vi "Number Widget.vi"(8 "Error In":errorcluster, 11 "Post-Bundled Subclass":refnum<class "4. Number Widget.lvclass">) -> (0 "Error Out":errorcluster, 3 "New Number Widget":refnum<class "4. Number Widget.lvclass">)   [LabVIEW 2013, in "4. Number Widget.lvclass"]
doc: "Copyright (c) 2016 Sze Howe Koh\nThis code is licensed under the MIT license"
uses:
  4. Number Widget.lvclass
  src/LabVIEW/Qt Widgets/QBoxLayout/Direction.ctl
  src/LabVIEW/Qt Widgets/QFrame/Shadow.ctl
  src/LabVIEW/Qt Widgets/QFrame/Shape.ctl
  4. Number Widget.lvclass/4. Number Widget.ctl
  src/LabVIEW/LQ Core/LQCoreEngine/_Polymorphic Instances/Connect_SignatureIn_QtSlot.vi
  src/LabVIEW/Qt Widgets/QFrame/setFrameShadow.vi
  src/LabVIEW/Qt Widgets/QFrame/setFrameShape.vi
  src/LabVIEW/Qt Widgets/QLCDNumber/QLCDNumber.lvclass
  src/LabVIEW/Qwt/QwtSlider/QwtSlider.lvclass
  src/LabVIEW/Qt Widgets/QBoxLayout/QBoxLayout.lvclass
  src/LabVIEW/Qt Widgets/QWidget/QWidget.lvclass
  src/LabVIEW/LQ Core/LQCoreEngine/LQCoreEngine.lvclass
  src/LabVIEW/Qt Widgets/QFrame/QFrame.lvclass
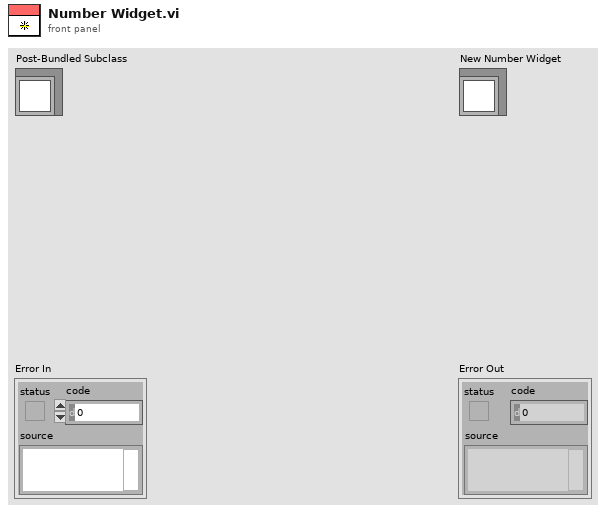
[diagram p1: front panel]
types:
  T1 = typedef "QFrame.lvclass/Shape.ctl" = i32
  T2 = typedef "QFrame.lvclass/Shadow.ctl" = i32
  T3 = typedef "QBoxLayout.lvclass/Direction.ctl" = i32
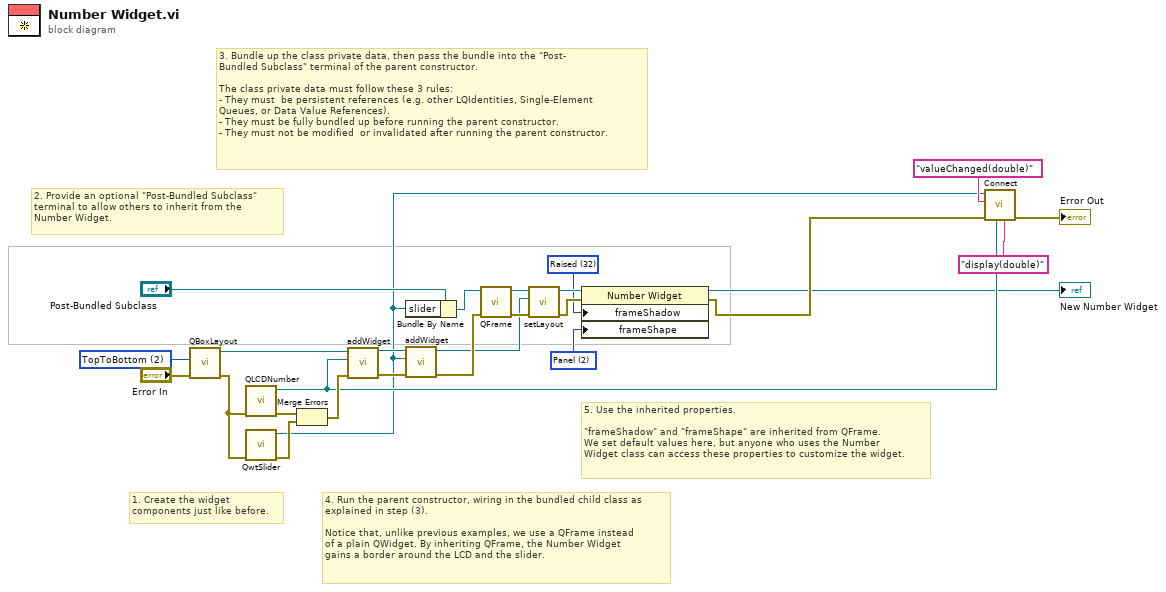
[diagram p0: block diagram]
diagram:
  w1 = T1 2 items=["NoFrame", "Box", "Panel", "HLine", "VLine", "StyledPanel"] ("frameShape")
  w2 = T2 32 items=["Plain"=16, "Raised"=32, "Sunken"=48] ("frameShadow")
  w7 = T3 2 items=["LeftToRight", "RightToLeft", "TopToBottom", "BottomToTop"] ("direction")
  # "1. Create the widget\ncomponents just like before."
  # "2. Provide an optional \"Post-Bundled Subclass\"\nterminal to allow others to inherit from the\nNumber Widget."
  # "5. Use the inherited properties.\n\n\"frameShadow\" and \"frameShape\" are inherited from QFrame.\nWe set default values here, but anyone who uses the Number\nWidget class can access these properties to customize the widget."
  # "4. Run the parent constructor, wiring in the bundled child class as\nexplained in step (3).\n\nNotice that, unlike previous examples, we use a QFrame instead\nof a plain QWidget. By inheriting QFrame, the Number Widget\ngains a border around the LCD and the slider."
  # "3. Bundle up the class private data, then pass the bundle into the \"Post-\nBundled Subclass\" terminal of the parent constructor.\n\nThe class private data must follow these 3 rules:\n- They must  be persistent references (e.g. other LQIdentities, Single-Element\nQueues, or Data Value References).\n- They must be fully bundled up before running the parent constructor.\n- They must not be modified  or invalidated after running the parent constructor."
  n1 = call "QBoxLayout.vi"("Error In"="Error In", "direction"=w7) -> ("Error Out"=w14:errorcluster, "New QBoxLayout"=w22:refnum<class "QBoxLayout.lvclass">)  [unwired: 8 in]
  n2 = call "QLCDNumber.vi"("Error In"=w14) -> ("Error Out"=w12:errorcluster, "New QLCDNumber"=w11:refnum<class "QLCDNumber.lvclass">)  [unwired: 9 in]
  n3 = call "QwtSlider.vi"("Error In"=w14) -> ("Error Out"=w13:errorcluster, "New QwtSlider"=w8:refnum<class "QwtSlider.lvclass">)  [unwired: 9 in]
  n4 = Merge Errors(w12, w13) -> (w23:errorcluster)
  n5 = call "addWidget.vi"("Error In"=w23, "widget"=w11, "QBoxLayout In"=w22) -> ("Error Out"=w18:errorcluster, "QBoxLayout Out"=w21:refnum<class "QBoxLayout.lvclass">)  [unwired: 7 in]
  n6 = Bundle By Name(cluster="Post-Bundled Subclass", "slider"=w8) -> (w6:refnum<class "4. Number Widget.lvclass">)
  n7 = call "addWidget.vi"("Error In"=w18, "widget"=w8, "QBoxLayout In"=w21) -> ("Error Out"=w25:errorcluster, "QBoxLayout Out"=w19:refnum<class "QBoxLayout.lvclass">)  [unwired: 7 in]
  n8 = call "QFrame.vi"("Error In"=w25, "Post-Bundled Subclass"=w6) -> ("Error Out"=w24:errorcluster, "New QFrame"=w20:refnum<class "4. Number Widget.lvclass">)  [unwired: 8 in]
  n9 = call "setLayout.vi"("Error In"=w24, "layout"=w19, "QWidget In"=w20) -> ("Error Out"=w3:errorcluster, "QWidget Out"=w5:refnum<class "4. Number Widget.lvclass">)  [unwired: 7 in]
  n10 = property class="Number Widget"(reference=w5, error in=w3, "frameShadow"=w2, "frameShape"=w1) -> (reference out=→"New Number Widget":refnum<class "4. Number Widget.lvclass">, error out=w26:errorcluster)
  n11 = call-poly "Connect.vi"("Slot Signature"="display(double)" ("Slot"), "Receiver"=w11, "Error In"=w26, "Signal Signature"="valueChanged(double)" ("Signal"), "Sender In"=w8) -> ("Error Out"=→"Error Out":errorcluster)  [unwired: 5 in, 1 out]
